vi "Input Channel Page.vi"(8 "error in (no error)":errorcluster, 11 "Node Ptr":T1 format="%.0x") -> (0 "error out":errorcluster)   [LabVIEW 2011, in "Interpolate 1D Array Custom Device.lvlib"]
uses:
  Interpolate 1D Array Custom Device.lvlib
  <vilib>/NI Veristand/Custom Device API/Custom Device Item Ref.ctl
  <vilib>/NI Veristand/Custom Device API/Custom Device API.lvlib
panel:
  in  "Default Value":dbl
  in  "Header":cluster{"Section Name":string}={"Section Name"="Custom Device Item Settings"}
  in  "Description":string
  in  "Name":string
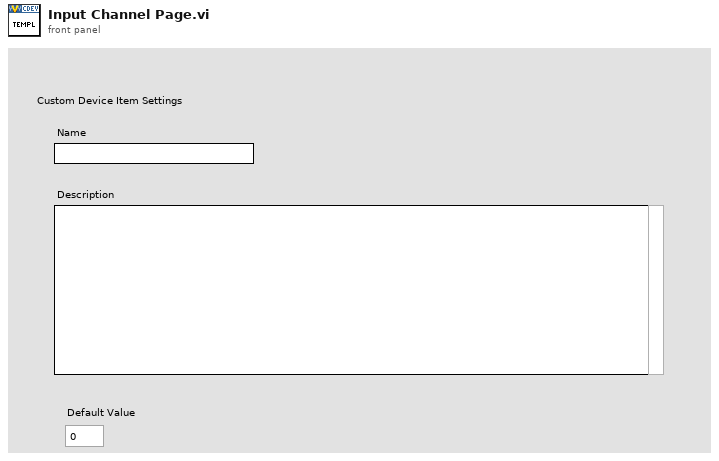
[diagram p1: front panel]
types:
  T1 = typedef "Custom Device API.lvlib/Custom Device Item Ref.ctl" = u64
  T2 = typedef "Custom Device API.lvlib/Custom Device Channel.ctl" = cluster{"Type":T3, "Units":string, "Default Value":dbl, "Faultable":bool, "Scalable":bool}
  T3 = typedef "Custom Device API.lvlib/Custom Device Channel Type.ctl" = enum16{"Input", "Output"}
  T4 = typedef "Custom Device API.lvlib/Custom Device Item Info.ctl" = cluster{"Name":string, "Is Channel":bool, "GUID":string}
  T5 = typedef "Custom Device API.lvlib/Custom Device Commands.ctl" = enum16{"Default", "Item renamed", "Shutdown", "Dynamic button pressed"}
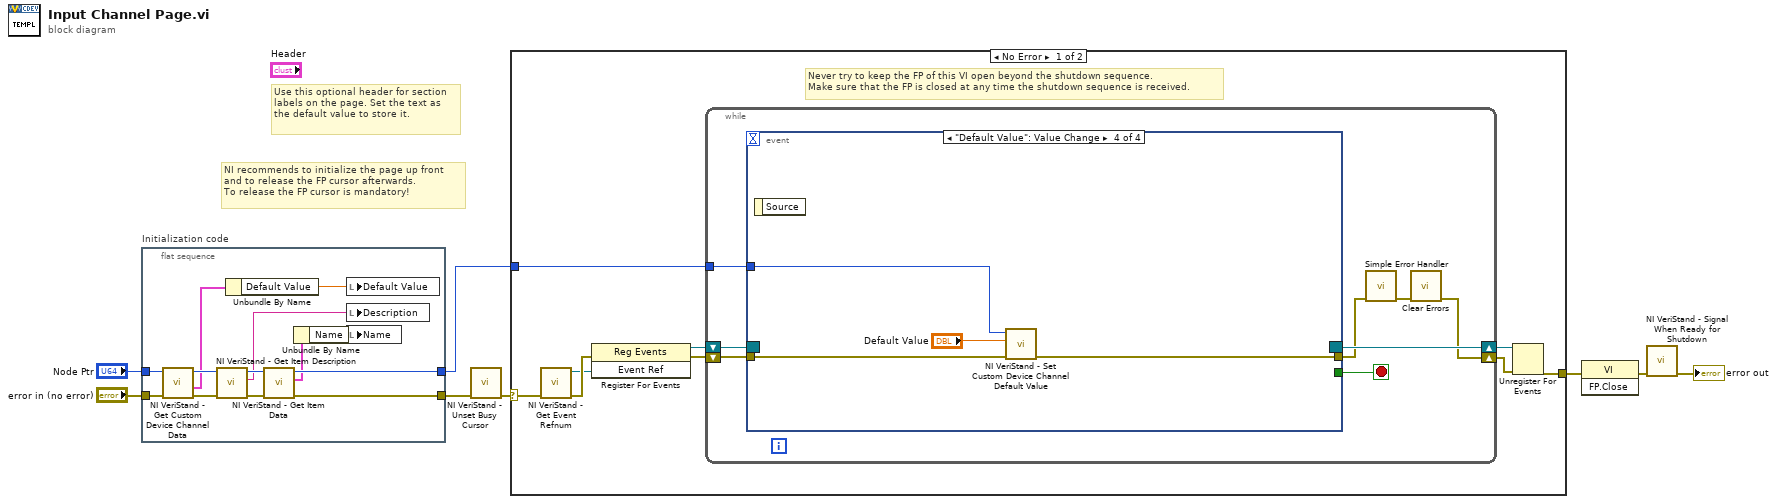
[diagram p0: block diagram]
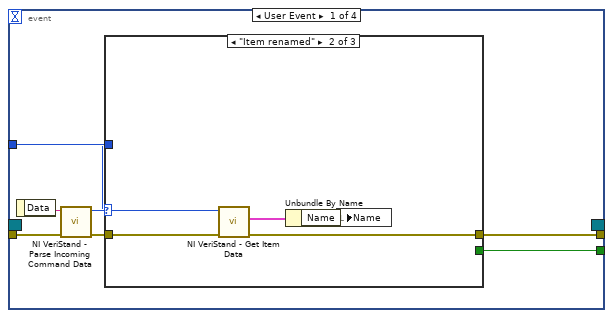
[diagram p2: hidden frame]
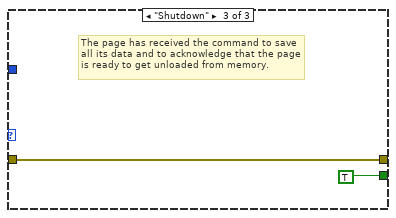
[diagram p4: hidden frame]
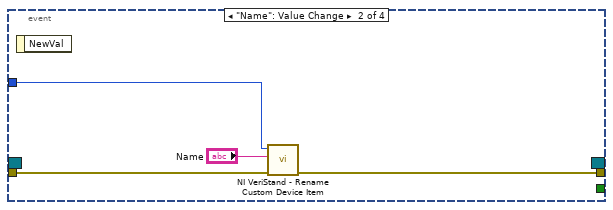
[diagram p5: hidden frame]
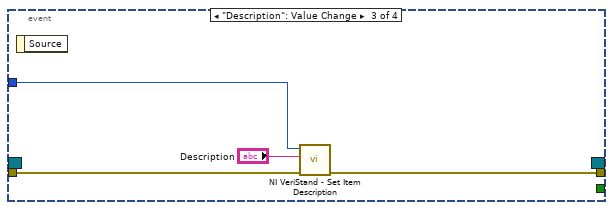
[diagram p6: hidden frame]
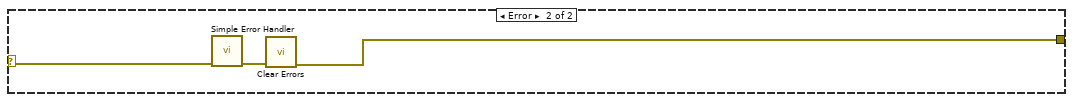
[diagram p7: hidden frame]
diagram:
  # "Use this optional header for section labels on the page. Set the text as the default value to store it."
  # "NI recommends to initialize the page up front\nand to release the FP cursor afterwards.\nTo release the FP cursor is mandatory!"
  n1 = flat-sequence "Initialization code" {
    tunnel: "error in (no error)" -> [w11]
    tunnel: "Node Ptr" -> [w14]
    tunnel: [w16] -> w4
    tunnel: [w21] -> w1
    frame #0 {
      n2 = call <vilib>:"NI VeriStand - Get Custom Device Channel Data.vi"("error in (no error)"=w11, "Channel Ref in"=w14) -> ("error out"=w12:errorcluster, "Channel"=w10:T2, "Channel Ref out"=w13:T1)  [unwired: 4 in, 3 out]
      n3 = call <vilib>:"NI VeriStand - Get Item Description.vi"("error in (no error)"=w12, "Item Ref in"=w13) -> ("error out"=w18:errorcluster, "Description"=w19:string, "Item Ref out"=w20:T1)  [unwired: 7 out]
      n4 = Unbundle By Name(w10) -> ("Default Value"=w9:dbl)
      n5 = call <vilib>:"NI VeriStand - Get Item Data.vi"("error in (no error)"=w18, "Item Ref in"=w20) -> ("error out"=w16:errorcluster, "Item Info"=w17:T4, "Item Ref out"=w21:T1)  [unwired: 7 out]
      n6 = Unbundle By Name(w17) -> ("Name"=w15:string)
      n7 = local write "Default Value"(w9) -> ()
      n8 = local write "Description"(w19) -> ()
      n9 = local write "Name"(w15) -> ()
    }
  }
  n10 = call <vilib>:"NI VeriStand - Unset Busy Cursor.vi"("error in (no error)"=w4) -> ("error out"=w3:errorcluster)  [unwired: 10 out]
  n11 = case shown="No Error" w3 {
    selector: w3 -> [w22 w68]
    tunnel: [w27 w66] -> w8
    tunnel: w1 -> [w23 _]
    frame No Error {
      # "Never try to keep the FP of this VI open beyond the shutdown sequence.\nMake sure that the FP is closed at any time the shutdown sequence is received."
      n12 = call <vilib>:"NI VeriStand - Get Event Refnum.vi"("error in (no error)"=w22) -> ("error out"=w30:errorcluster, "Event Ref"=w26:refnum<user-event>)  [unwired: 9 out]
      n13 = register-events(error in=w30, w26) -> (reference out=w24:refnum<event-registration>, error out=w25:errorcluster)  [unwired: 1 in]
      n14 = while {
        tunnel: w23 -> [w34]
        shift-right: [w31] -> w28
        shift-left: w25 -> [w37]
        shift-right: [w38] -> w29
        shift-left: w24 -> [w36]
        stop <- w35 stop-if-true
        n15 = event shown="[3] \"Default Value\": Value Change" {
          selector: w36 -> [_ _ _ _]
          dyn-events: [_ _ _ _] -> w38
          timeout: _ -> [_ _ _ _]
          tunnel: w37 -> [w45 w57 w60 w64]
          tunnel: [w41 _ _ _] -> w35
          tunnel: [w40 w56 w59 w63] -> w33
          tunnel: w34 -> [w39 w55 w61 w65]
          event User Event {
            n16 = event-data() -> ("Data"=w44:string)  [unwired: 1 out]
            n17 = call <vilib>:"NI VeriStand - Parse Incoming Command Data.vi"("error in (no error)"=w45, "Incoming data"=w44) -> ("error out"=w43:errorcluster, "Action"=w42:T5)  [unwired: 8 out]
            n18 = case shown="\"Item renamed\"" w42 {
              tunnel: w43 -> [w46 w51 w52]
              tunnel: [_ _ TRUE] -> w41
              tunnel: [w46 w48 w52] -> w40
              tunnel: w39 -> [_ w50 _]
              frame "Default", Default {
              }
              frame "Item renamed" {
                n19 = call <vilib>:"NI VeriStand - Get Item Data.vi"("error in (no error)"=w51, "Item Ref in"=w50) -> ("error out"=w48:errorcluster, "Item Info"=w49:T4)  [unwired: 8 out]
                n20 = Unbundle By Name(w49) -> ("Name"=w47:string)
                n21 = local write "Name"(w47) -> ()
              }
              frame "Shutdown" {
                # "The page has received the command to save all its data and to acknowledge that the page is ready to get unloaded from memory."
              }
            }
          }
          event "Name": Value Change {
            n22 = event-data() -> ()  [unwired: 2 out]
            n23 = call <vilib>:"NI VeriStand - Rename Custom Device Item.vi"("error in (no error)"=w57, "New Name"="Name", "Item Ref in"=w55) -> ("error out"=w56:errorcluster)  [unwired: 8 out]
          }
          event "Description": Value Change {
            n24 = event-data() -> ()  [unwired: 2 out]
            n25 = call <vilib>:"NI VeriStand - Set Item Description.vi"("error in (no error)"=w60, "Description"="Description", "Item Ref in"=w61) -> ("error out"=w59:errorcluster)  [unwired: 8 out]
          }
          event "Default Value": Value Change {
            n26 = event-data() -> ()  [unwired: 2 out]
            n27 = call <vilib>:"NI VeriStand - Set Custom Device Channel Default Value.vi"("error in (no error)"=w64, "Default Value"="Default Value", "Channel Ref in"=w65) -> ("error out"=w63:errorcluster)  [unwired: 7 in, 1 out]
          }
        }
        n28 = call <vilib>:"Simple Error Handler.vi"("error in (no error)"=w33) -> ("error out"=w32:errorcluster)  [unwired: 1 in, 7 out]
        n29 = call <vilib>:"Clear Errors.vi"("error in (no error)"=w32) -> ("error out"=w31:errorcluster)  [unwired: 6 out]
      }
      n30 = Unregister For Events(event registration refnum=w29, error in=w28) -> (error out=w27:errorcluster)
    }
    frame Error {
      n31 = call <vilib>:"Simple Error Handler.vi"("error in (no error)"=w68) -> ("error out"=w67:errorcluster)  [unwired: 1 in, 7 out]
      n32 = call <vilib>:"Clear Errors.vi"("error in (no error)"=w67) -> ("error out"=w66:errorcluster)  [unwired: 6 out]
    }
  }
  n33 = invoke class="VI" method="FP.Close"(error in=w8) -> (error out=w7:errorcluster)  [unwired: 2 in, 2 out]
  n34 = call <vilib>:"NI VeriStand - Signal When Ready for Shutdown.vi"("error in (no error)"=w7) -> ("error out"=→"error out":errorcluster)  [unwired: 10 out]
